vi "Test CSV reader.vi"() -> ()   [LabVIEW 2017]
uses:
  CSV Reader/Mode CSV reader.ctl
panel:
  out "Timestamps 4":timestamp[](array[timestamp])
  out "Complex 4":cdb[][](array[numeric])
  out "Analog 4":dbl[][](array[numeric])
  out "EOF? 4":bool
  out "Timestamps 3":timestamp[](array[timestamp])
  out "Complex 3":cdb[][](array[numeric])
  out "Analog 3":dbl[][](array[numeric])
  out "EOF? 3":bool
  out "Timestamps 2":timestamp[](array[timestamp])
  out "Complex 2":cdb[][](array[numeric])
  out "Analog 2":dbl[][](array[numeric])
  out "EOF? 2":bool
  out "EOF?":bool
  out "Analog":dbl[][](array[numeric])
  out "Complex":cdb[][](array[numeric])
  out "Timestamps":timestamp[](array[timestamp])
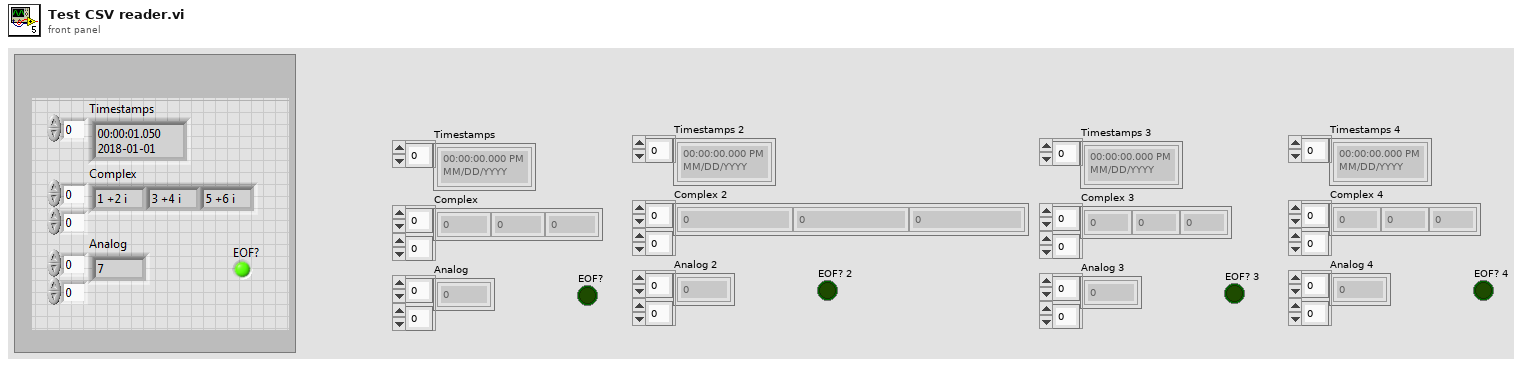
[diagram p1: front panel]
types:
  T1 = typedef "Mode CSV reader.ctl" = enum16{"Full timestamp", "Relative Time", "Seconds Time"}
  T2 = cluster{"Mode":T1, "delimiter (\\t)":string, "Path":path, "Rectangular?":bool}
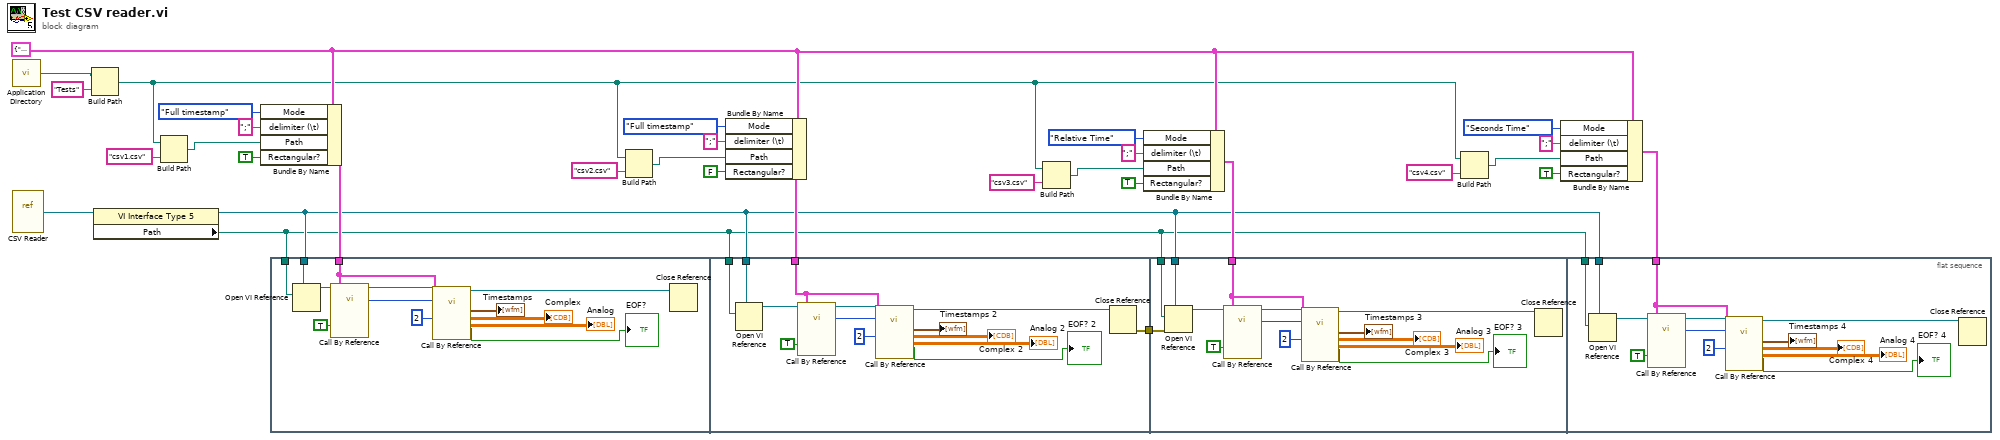
[diagram p0: block diagram]
diagram:
  w3 = T2 {"Mode"=enum."Full timestamp", "delimiter (\\t)"="", "Path"=path "", "Rectangular?"=FALSE} ("Config CSV")
  n1 = call <vilib>:"Application Directory.vi"() -> ("Application Directory"=w27:path)
  n2 = vi-ref "CSV Reader.vi"() -> (w18:refnum<vi>)
  n3 = Build Path(base path=w27, name or relative path="Tests") -> (appended path=w1:path)
  n4 = property class="VI Interface Type 5"(reference=w18) -> (reference out=w10:refnum<vi>, "Path"=w9:path)  [unwired: 1 in, 1 out]
  n5 = Build Path(base path=w1, name or relative path="csv1.csv") -> (appended path=w29:path)
  n6 = Bundle By Name(cluster=w3, "Mode"=Mode_CSV_reader."Full timestamp", "delimiter (\\t)"=";" ("delimiter (\\t)"), "Path"=w29, "Rectangular?"=TRUE) -> (w25:T2)
  n7 = flat-sequence {
    tunnel: w10 -> [w44]
    tunnel: w9 -> [w43]
    tunnel: w25 -> [w36]
    tunnel: w10 -> [w50]
    tunnel: w9 -> [w49]
    tunnel: w19 -> [w48]
    tunnel: [w46] -> w17
    tunnel: w17 -> [w63]
    tunnel: w11 -> [w62]
    tunnel: w10 -> [w61]
    tunnel: w9 -> [w60]
    tunnel: w10 -> [w76]
    tunnel: w9 -> [w75]
    tunnel: w2 -> [w74]
    frame #0 {
      n8 = Open VI Reference(type specifier VI Refnum (for type only)=w44, vi path=w43) -> (vi reference=w45:refnum<vi>)  [unwired: 4 in, 1 out]
      n9 = call-by-ref "?"(reference=w45, "Reset"=TRUE, "Config CSV"=w36) -> (reference out=w42:refnum<vi>, "Index out"=w37:i32)  [unwired: 6 in, 5 out]
      n10 = call-by-ref "?"(reference=w42, "Index in"=w37, "Parcel Length"=2, "Config CSV"=w36) -> (reference out=w34:refnum<vi>, "Analog"=→"Analog":dbl[][], "Complex"=→"Complex":cdb[][], "Timestamps"=→"Timestamps":timestamp[], "EOF?"=→"EOF?":bool)  [unwired: 5 in, 2 out]
      n11 = Close Reference(reference=w34) -> ()  [unwired: 1 in, 1 out]
    }
    frame #1 {
      n12 = Open VI Reference(type specifier VI Refnum (for type only)=w50, vi path=w49) -> (vi reference=w51:refnum<vi>)  [unwired: 4 in, 1 out]
      n13 = call-by-ref "?"(reference=w51, "Reset"=TRUE, "Config CSV"=w48) -> (reference out=w52:refnum<vi>, "Index out"=w57:i32)  [unwired: 6 in, 5 out]
      n14 = call-by-ref "?"(reference=w52, "Index in"=w57, "Parcel Length"=2, "Config CSV"=w48) -> (reference out=w59:refnum<vi>, "Analog"=→"Analog 2":dbl[][], "Complex"=→"Complex 2":cdb[][], "Timestamps"=→"Timestamps 2":timestamp[], "EOF?"=→"EOF? 2":bool)  [unwired: 5 in, 2 out]
      n15 = Close Reference(reference=w59) -> (error out=w46:errorcluster)  [unwired: 1 in]
    }
    frame #2 {
      n16 = Open VI Reference(type specifier VI Refnum (for type only)=w61, vi path=w60, error in (no error)=w63) -> (vi reference=w72:refnum<vi>)  [unwired: 3 in, 1 out]
      n17 = call-by-ref "?"(reference=w72, "Reset"=TRUE, "Config CSV"=w62) -> (reference out=w71:refnum<vi>, "Index out"=w66:i32)  [unwired: 6 in, 5 out]
      n18 = call-by-ref "?"(reference=w71, "Index in"=w66, "Parcel Length"=2, "Config CSV"=w62) -> (reference out=w64:refnum<vi>, "Analog"=→"Analog 3":dbl[][], "Complex"=→"Complex 3":cdb[][], "Timestamps"=→"Timestamps 3":timestamp[], "EOF?"=→"EOF? 3":bool)  [unwired: 5 in, 2 out]
      n19 = Close Reference(reference=w64) -> ()  [unwired: 1 in, 1 out]
    }
    frame #3 {
      n20 = Open VI Reference(type specifier VI Refnum (for type only)=w76, vi path=w75) -> (vi reference=w78:refnum<vi>)  [unwired: 4 in, 1 out]
      n21 = call-by-ref "?"(reference=w78, "Reset"=TRUE, "Config CSV"=w74) -> (reference out=w79:refnum<vi>, "Index out"=w84:i32)  [unwired: 6 in, 5 out]
      n22 = call-by-ref "?"(reference=w79, "Index in"=w84, "Parcel Length"=2, "Config CSV"=w74) -> (reference out=w86:refnum<vi>, "Analog"=→"Analog 4":dbl[][], "Complex"=→"Complex 4":cdb[][], "Timestamps"=→"Timestamps 4":timestamp[], "EOF?"=→"EOF? 4":bool)  [unwired: 5 in, 2 out]
      n23 = Close Reference(reference=w86) -> ()  [unwired: 1 in, 1 out]
    }
  }
  n24 = Build Path(base path=w1, name or relative path="csv2.csv") -> (appended path=w23:path)
  n25 = Bundle By Name(cluster=w3, "Mode"=Mode_CSV_reader."Full timestamp", "delimiter (\\t)"=";" ("delimiter (\\t)"), "Path"=w23, "Rectangular?"=FALSE) -> (w19:T2)
  n26 = Build Path(base path=w1, name or relative path="csv3.csv") -> (appended path=w13:path)
  n27 = Bundle By Name(cluster=w3, "Mode"=Mode_CSV_reader."Relative Time", "delimiter (\\t)"=";" ("delimiter (\\t)"), "Path"=w13, "Rectangular?"=TRUE) -> (w11:T2)
  n28 = Build Path(base path=w1, name or relative path="csv4.csv") -> (appended path=w7:path)
  n29 = Bundle By Name(cluster=w3, "Mode"=Mode_CSV_reader."Seconds Time", "delimiter (\\t)"=";" ("delimiter (\\t)"), "Path"=w7, "Rectangular?"=TRUE) -> (w2:T2)
